vi "PH_DataViewer.set PU GUI Elements.vi"(0 "index":i32, 2 "PP PUs Vers 1":T3[](array[typedef]) {"State" items=["no info", "off/false/out", "on/true/in", "Failure", "Alarm", "Status 1", "Status 2", "Status 3"]}, 4 "PP PUs Vers 2":T1[](array[typedef]) {"State" items=["no info", "off/false/out", "on/true/in", "Failure", "Alarm", "Status 1", "Status 2", "Status 3"]}, 7 "Version":u8) -> (10 "Instances":string[](array[string]), 12 "index":i32, 13 "PP PUs":T3[](array[typedef]) {"State" items=["no info", "off/false/out", "on/true/in", "Failure", "Alarm", "Status 1", "Status 2", "Status 3"]}, 14 "Snapshot: Date before Shot":string, 15 "State after Shot":T2 caption="PPMA Sequencer State" items=["no info", "off/false/out", "on/true/in", "Failure", "Alarm", "Status 1", "Status 2", "Status 3"], 16 "Snapshot: Time before Shot":string, 17 "PU in use after Shot":bool, 18 "PU in use before Shot":bool, 19 "Snapshot: Time after Shot":string, 20 "State before Shot":T2 caption="PPMA Sequencer State" items=["no info", "off/false/out", "on/true/in", "Failure", "Alarm", "Status 1", "Status 2", "Status 3"], 21 "Waiting Time over?":bool, 22 "Voltage [V]":dbl, 23 "Delay [s]":dbl, 24 "Gate Gen Channel":string, 25 "Timeout SM":string, 26 "Time betweeen Shots [Min]":dbl, 27 "Snapshot: Date after Shot":string)   [LabVIEW 2014, in "PH_DataViewer.lvlib"]
doc: "This VI prepares the information to be indicated."
uses:
  PH_DataViewer.lvlib
  PH_Common.PP PU Data.ctl
  PH_Basics/PH_StatusHandler/PH_StatusHandler.Status.ctl
  PH_Common.PP PU Data Vers2.ctl
  PH_Basics/PH_StatusHandler/PH_StatusHandler.lvlib
  PH_Basics/PH_Common/PH_Common.lvlib
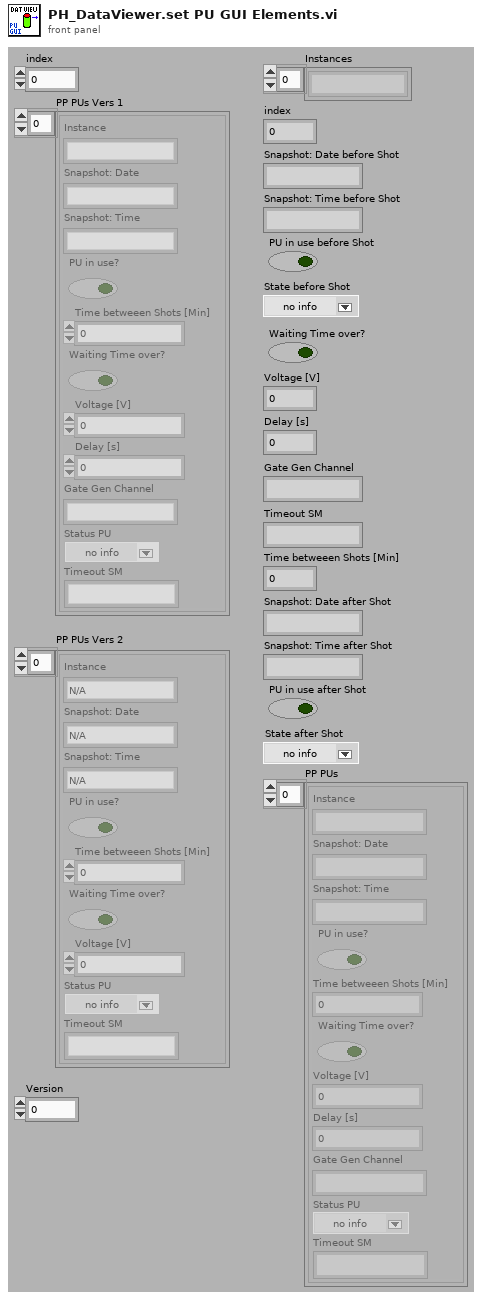
[diagram p1: front panel]
types:
  T1 = typedef "PH_DataViewer.lvlib/PH_Common.PP PU Data Vers2.ctl" = cluster{"Instance":string, "Snapshot: Date":string, "Snapshot: Time":string, "PU in use?":bool, "Time betweeen Shots [Min]":dbl, "Waiting Time over?":bool, "Voltage [V]":dbl, "State":T2, "Timeout SM":string}
  T2 = typedef "PH_StatusHandler.lvlib/PH_StatusHandler.Status.ctl" = i16
  T3 = typedef "PH_DataViewer.lvlib/PH_Common.PP PU Data.ctl" = cluster{"Instance":string, "Snapshot: Date":string, "Snapshot: Time":string, "PU in use?":bool, "Time betweeen Shots [Min]":dbl, "Waiting Time over?":bool, "Voltage [V]":dbl, "Delay [s]":dbl, "Gate Gen Channel":string, "State":T2, "Timeout SM":string}
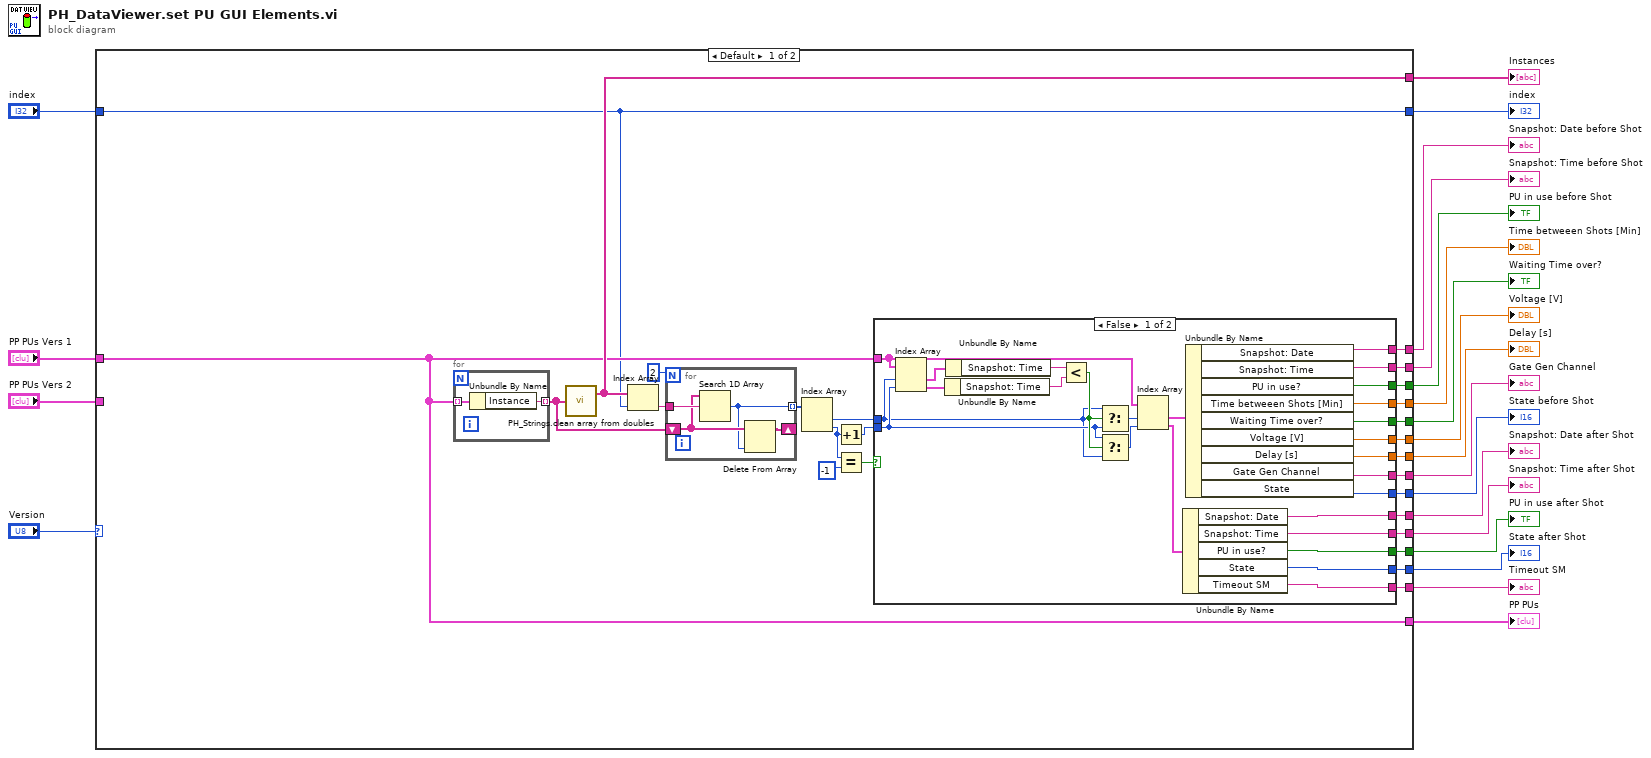
[diagram p0: block diagram]
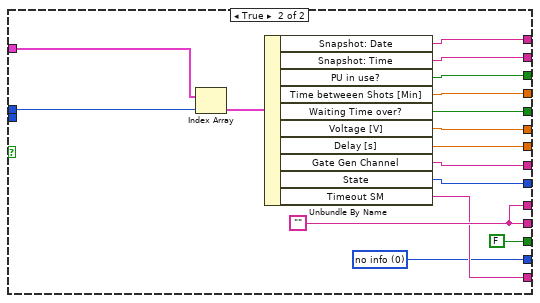
[diagram p2: hidden frame]
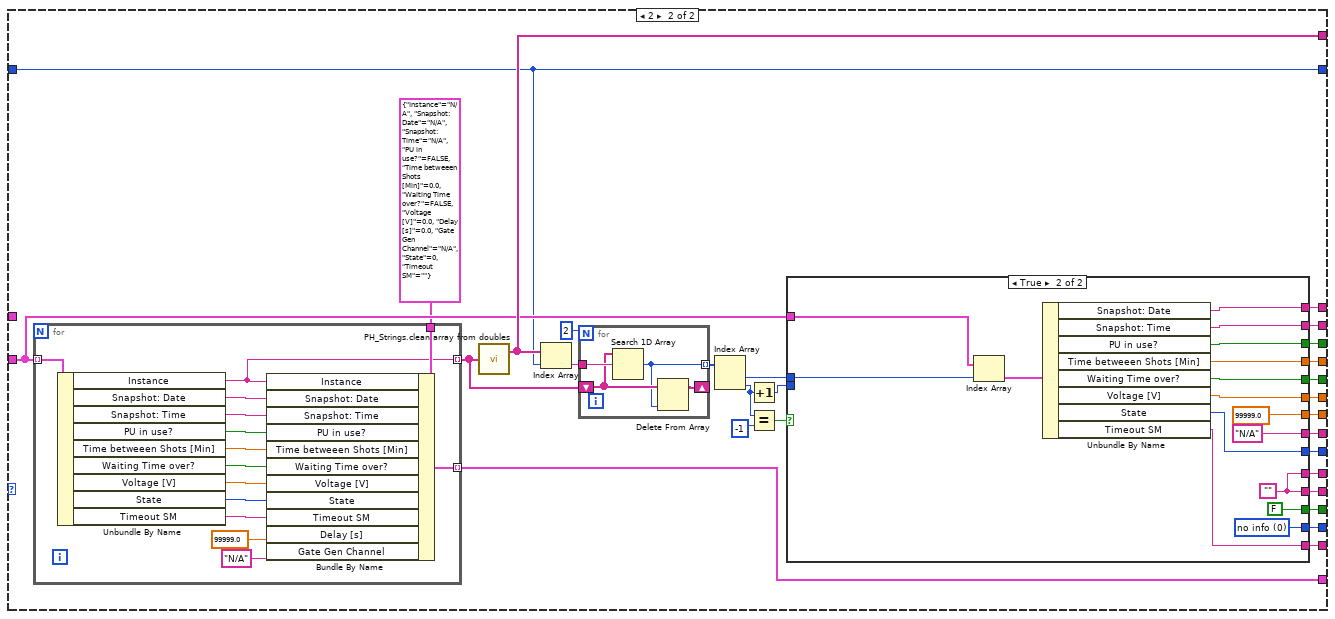
[diagram p3: hidden frame]
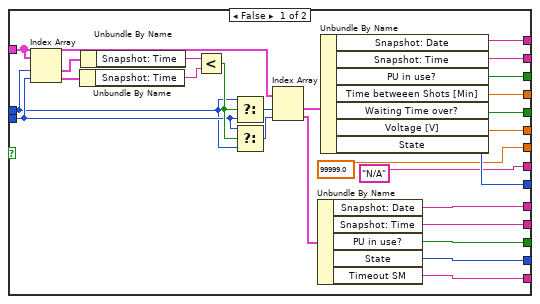
[diagram p4: hidden frame]
diagram:
  n1 = case shown="Default" "Version" {
    tunnel: [w47 w123] -> w21
    tunnel: [w46 w122] -> w20
    tunnel: [w45 w121] -> w19
    tunnel: [w44 w120] -> w18
    tunnel: [w43 w119] -> w17
    tunnel: [w42 w118] -> w16
    tunnel: [w41 w117] -> w15
    tunnel: [w40 w116] -> w14
    tunnel: [w39 w115] -> w13
    tunnel: [w38 w114] -> w12
    tunnel: [w37 w113] -> w11
    tunnel: [w36 w112] -> w10
    tunnel: [w35 w111] -> w9
    tunnel: [w32 w108] -> w8
    tunnel: [w22 w96] -> w7
    tunnel: [w26 w102] -> w6
    tunnel: "PP PUs Vers 1" -> [w23 _]
    tunnel: [w23 w97] -> w3
    tunnel: "PP PUs Vers 2" -> [_ w99]
    tunnel: "index" -> [w22 w96]
    frame Default {
      n2 = for {
        tunnel: w23 -> [w49] mode=indexing
        tunnel: [w48] -> w24 mode=indexing
        n3 = Unbundle By Name(w49) -> ("Instance"=w48:string)
      }
      n4 = call "PH_Strings.clean array from doubles.vi"("Array Input"=w24) -> ("Array Output"=w26:string[])  [unwired: 1 out]
      n5 = Index Array(array=w26, index=w22) -> (element=w25:string)
      n6 = for {
        N: 2 -> [_]
        tunnel: w25 -> [w95]
        tunnel: [w93] -> w30 mode=indexing
        shift-right: [w92] -> _
        shift-left: w24 -> [w94]
        n7 = Search 1D Array(1D array=w94, element=w95) -> (index of element=w93:i32)  [unwired: 1 in]
        n8 = Delete From Array(array=w94, index=w93) -> (array with subset deleted=w92:string[])  [unwired: 1 in, 1 out]
      }
      n9 = Index Array(array=w30) -> (element #1=w31:i32, element #2=w33:i32)  [unwired: 2 in]
      n10 = Increment(x=w33) -> (x+1=w34:i32)
      n11 = Equal?(x=w33, y=-1 ("index of element")) -> (x = y?=w29:bool)
      n12 = case shown="False" w29 {
        tunnel: w23 -> [w71 w91]
        tunnel: w34 -> [w68 _]
        tunnel: w31 -> [w66 w80]
        tunnel: [w63 w88] -> w32
        tunnel: [w64 w89] -> w35
        tunnel: [w62 w87] -> w36
        tunnel: [w61 w86] -> w37
        tunnel: [w60 w85] -> w38
        tunnel: [w59 w84] -> w39
        tunnel: [w58 w83] -> w40
        tunnel: [w57 w82] -> w41
        tunnel: [w56 w81] -> w42
        tunnel: [w54 w79] -> w44
        tunnel: [w53 w79] -> w43
        tunnel: [w52 FALSE ("PU in use?")] -> w45
        tunnel: [w51 w77] -> w46
        tunnel: [w50 w78] -> w47
        frame False {
          n13 = Index Array(array=w71, index #1=w66, index #2=w68) -> (element #1=w74:T3, element #2=w75:T3)
          n14 = Unbundle By Name(w75) -> ("Snapshot: Time"=w72:string)
          n15 = Unbundle By Name(w74) -> ("Snapshot: Time"=w73:string)
          n16 = Less?(x=w73, y=w72) -> (x < y?=w69:bool)
          n17 = Select(t=w66, s=w69, f=w68) -> (s? t:f=w70:i32)
          n18 = Select(t=w68, s=w69, f=w66) -> (s? t:f=w67:i32)
          n19 = Index Array(array=w71, index #1=w70, index #2=w67) -> (element #1=w65:T3, element #2=w55:T3)
          n20 = Unbundle By Name(w55) -> ("Snapshot: Date"=w54:string, "Snapshot: Time"=w53:string, "PU in use?"=w52:bool, "State"=w51:T2, "Timeout SM"=w50:string)
          n21 = Unbundle By Name(w65) -> ("Snapshot: Date"=w64:string, "Snapshot: Time"=w63:string, "PU in use?"=w62:bool, "Time betweeen Shots [Min]"=w61:dbl, "Waiting Time over?"=w60:bool, "Voltage [V]"=w59:dbl, "Delay [s]"=w58:dbl, "Gate Gen Channel"=w57:string, "State"=w56:T2)
        }
        frame True {
          w77 = T2 0 items=["no info", "off/false/out", "on/true/in", "Failure", "Alarm", "Status 1", "Status 2", "Status 3"] ("State")
          w79 = ""
          n22 = Index Array(array=w91, index=w80) -> (element=w90:T3)
          n23 = Unbundle By Name(w90) -> ("Snapshot: Date"=w89:string, "Snapshot: Time"=w88:string, "PU in use?"=w87:bool, "Time betweeen Shots [Min]"=w86:dbl, "Waiting Time over?"=w85:bool, "Voltage [V]"=w84:dbl, "Delay [s]"=w83:dbl, "Gate Gen Channel"=w82:string, "State"=w81:T2, "Timeout SM"=w78:string)
        }
      }
    }
    frame 2 {
      n24 = for {
        tunnel: w99 -> [w137] mode=indexing
        tunnel: [w135] -> w100 mode=indexing
        tunnel: T3 {"Instance"="N/A", "Snapshot: Date"="N/A", "Snapshot: Time"="N/A", "PU in use?"=FALSE, "Time betweeen Shots [Min]"=0.0, "Waiting Time over?"=FALSE, "Voltage [V]"=0.0, "Delay [s]"=0.0, "Gate Gen Channel"="N/A", "State"=0, "Timeout SM"=""} ("PPMA PU Data") -> [w136]
        tunnel: [w124] -> w97 mode=indexing
        n25 = Unbundle By Name(w137) -> ("Instance"=w135:string, "Snapshot: Date"=w134:string, "Snapshot: Time"=w133:string, "PU in use?"=w132:bool, "Time betweeen Shots [Min]"=w131:dbl, "Waiting Time over?"=w130:bool, "Voltage [V]"=w129:dbl, "State"=w128:T2, "Timeout SM"=w127:string)
        n26 = Bundle By Name(cluster=w136, "Instance"=w135, "Snapshot: Date"=w134, "Snapshot: Time"=w133, "PU in use?"=w132, "Time betweeen Shots [Min]"=w131, "Waiting Time over?"=w130, "Voltage [V]"=w129, "State"=w128, "Timeout SM"=w127, "Delay [s]"=99999.0, "Gate Gen Channel"="N/A") -> (w124:T3)
      }
      n27 = call "PH_Strings.clean array from doubles.vi"("Array Input"=w100) -> ("Array Output"=w102:string[])  [unwired: 1 out]
      n28 = Index Array(array=w102, index=w96) -> (element=w101:string)
      n29 = for {
        N: 2 -> [_]
        tunnel: w101 -> [w183]
        tunnel: [w181] -> w106 mode=indexing
        shift-right: [w180] -> _
        shift-left: w100 -> [w182]
        n30 = Search 1D Array(1D array=w182, element=w183) -> (index of element=w181:i32)  [unwired: 1 in]
        n31 = Delete From Array(array=w182, index=w181) -> (array with subset deleted=w180:string[])  [unwired: 1 in, 1 out]
      }
      n32 = Index Array(array=w106) -> (element #1=w107:i32, element #2=w109:i32)  [unwired: 2 in]
      n33 = Increment(x=w109) -> (x+1=w110:i32)
      n34 = Equal?(x=w109, y=-1 ("index of element")) -> (x = y?=w105:bool)
      n35 = case shown="True" w105 {
        tunnel: w99 -> [w159 w179]
        tunnel: w110 -> [w156 _]
        tunnel: w107 -> [w154 w170]
        tunnel: [w151 w176] -> w108
        tunnel: [w152 w177] -> w111
        tunnel: [w150 w175] -> w112
        tunnel: [w149 w174] -> w113
        tunnel: [w148 w173] -> w114
        tunnel: [w147 w172] -> w115
        tunnel: [99999.0 ("Delay [s]") 99999.0 ("Delay [s]")] -> w116
        tunnel: ["N/A" ("Gate Gen Channel") "N/A" ("Gate Gen Channel")] -> w117
        tunnel: [w146 w171] -> w118
        tunnel: [w144 w169] -> w120
        tunnel: [w143 w169] -> w119
        tunnel: [w142 FALSE ("PU in use?")] -> w121
        tunnel: [w141 w167] -> w122
        tunnel: [w140 w168] -> w123
        frame False {
          n36 = Index Array(array=w159, index #1=w154, index #2=w156) -> (element #1=w162:T1, element #2=w163:T1)
          n37 = Unbundle By Name(w163) -> ("Snapshot: Time"=w160:string)
          n38 = Unbundle By Name(w162) -> ("Snapshot: Time"=w161:string)
          n39 = Less?(x=w161, y=w160) -> (x < y?=w157:bool)
          n40 = Select(t=w154, s=w157, f=w156) -> (s? t:f=w158:i32)
          n41 = Select(t=w156, s=w157, f=w154) -> (s? t:f=w155:i32)
          n42 = Index Array(array=w159, index #1=w158, index #2=w155) -> (element #1=w153:T1, element #2=w145:T1)
          n43 = Unbundle By Name(w145) -> ("Snapshot: Date"=w144:string, "Snapshot: Time"=w143:string, "PU in use?"=w142:bool, "State"=w141:T2, "Timeout SM"=w140:string)
          n44 = Unbundle By Name(w153) -> ("Snapshot: Date"=w152:string, "Snapshot: Time"=w151:string, "PU in use?"=w150:bool, "Time betweeen Shots [Min]"=w149:dbl, "Waiting Time over?"=w148:bool, "Voltage [V]"=w147:dbl, "State"=w146:T2)
        }
        frame True {
          w167 = T2 0 items=["no info", "off/false/out", "on/true/in", "Failure", "Alarm", "Status 1", "Status 2", "Status 3"] ("State")
          w169 = ""
          n45 = Index Array(array=w179, index=w170) -> (element=w178:T1)
          n46 = Unbundle By Name(w178) -> ("Snapshot: Date"=w177:string, "Snapshot: Time"=w176:string, "PU in use?"=w175:bool, "Time betweeen Shots [Min]"=w174:dbl, "Waiting Time over?"=w173:bool, "Voltage [V]"=w172:dbl, "State"=w171:T2, "Timeout SM"=w168:string)
        }
      }
    }
  }
  "Timeout SM" <- w21
  "State after Shot" <- w20
  "PU in use after Shot" <- w19
  "Snapshot: Date after Shot" <- w18
  "Snapshot: Time after Shot" <- w17
  "State before Shot" <- w16
  "Gate Gen Channel" <- w15
  "Delay [s]" <- w14
  "Voltage [V]" <- w13
  "Waiting Time over?" <- w12
  "Time betweeen Shots [Min]" <- w11
  "PU in use before Shot" <- w10
  "Snapshot: Date before Shot" <- w9
  "Snapshot: Time before Shot" <- w8
  "PP PUs" <- w3
  "Instances" <- w6
  "index" <- w7
